vi "PicoScope2000aExampleStreaming.vi"() -> ()   [LabVIEW 2016]
uses:
  Program Files/Pico Technology/SDK/lib/ps2000a.dll
  <vilib>/Waveform/DWDTOps.llb/DWDT Analog to Digital.vi
panel:
  out "Channel A":waveform(dbl)(graph)={"t0"=timestamp(0 s since 1904-01-01), "dt"=1.0000000130088963e-06, "Y"=array[49152 elements]}
  in  "Port 0 Settings":cluster{"Enabled":bool, "Logic Level":i16}={"Enabled"=FALSE, "Logic Level"=9830} {"Logic Level" items=["1.5V TTL"=9830, "2.5V CMOS"=16383]}
  out "Port 0":digitalwaveform(graph)={"t0"=timestamp(0 s since 1904-01-01), "dt"=1.0000000130088963e-06, "Y"={"transitions"=[], "data"=[]}}
  out "Sample Interval (sec)":dbl=1.0000000130088963e-06 format="%#.5p"
  out "Total Samples":u32=3096576 format="%#.6p"
  out "Triggered":bool
  out "TriggeredAt (Total samples)":u32 format="%#.6p"
  out "TriggeredAt (In Buffer)":u32 format="%#.6p"
  in  "Channel A Settings":T1={"Enabled"=TRUE, "Coupling"=1, "Range"=7, "Analogue Offset"=0.0} {"Range" items=["20 mV"=1, "50 mV"=2, "100 mV"=3, "200 mV"=4, "500 mV"=5, "1 V"=6, "2 V"=7, "5 V"=8, "10 V"=9, "20 V"=10]; "Coupling" items=["AC", "DC"]}
  in  "Trigger Settings":T2={"Trigger Enabled"=FALSE, "Trigger Source"=enum."Channel A", "Trigger Threshold (Volts)"=0.0, "Trigger Direction"=2, "Trigger Delay (samples)"=0, "Auto Trigger Time (ms)"=1000} {"Trigger Direction" items=["Rising"=2, "Falling"=3]}
  in  "Acquisition Settings":T3={"Auto Stop"=FALSE, "Desired Sample Interval"=1, "Pre-trigger Samples"=50000, "Post-trigger Samples"=50000, "Down-Sample Ratio"=1, "Down-Sample Mode"=0, "Overview Buffer Size"=1000000, "Time Units"=3} {"Time Units" items=["Nanoseconds (ns)"=2, "Microseconds (us)"=3, "Milliseconds (ms)"=4, "Seconds (s)"=5]; "Overview Buffer Size" format="%.0p"; "Down-Sample Mode" items=["None"=0, "Aggregate"=1, "Average"=2, "Decimate"=4, "Distribution"=8]; "Post-trigger Samples" format="%.0p"; "Pre-trigger Samples" format="%.0p"}
  in  "Apply Settings":bool
  in  "stop":bool
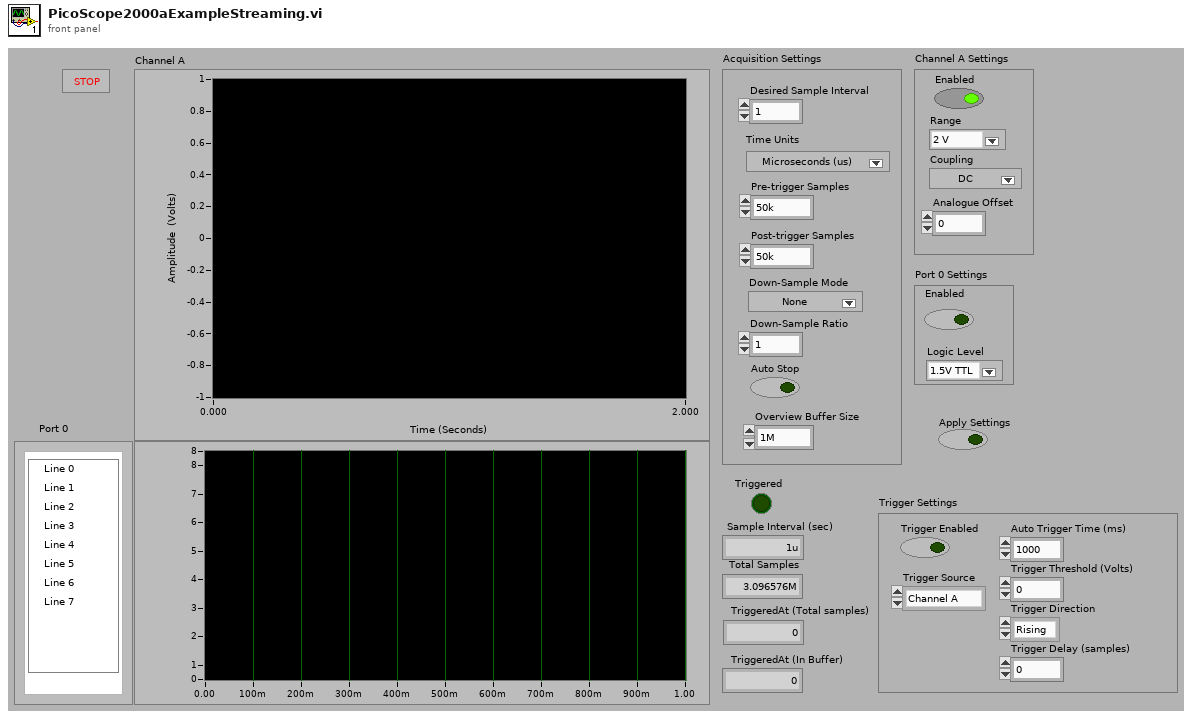
[diagram p1: front panel]
types:
  T1 = cluster{"Enabled":bool, "Coupling":i16, "Range":u16, "Analogue Offset":sgl}
  T2 = cluster{"Trigger Enabled":bool, "Trigger Source":enum16{"Channel A", "Channel B", "Channel C", "Channel D", "Ext."}, "Trigger Threshold (Volts)":dbl, "Trigger Direction":u16, "Trigger Delay (samples)":u32, "Auto Trigger Time (ms)":i16}
  T3 = cluster{"Auto Stop":bool, "Desired Sample Interval":u32, "Pre-trigger Samples":u32, "Post-trigger Samples":u32, "Down-Sample Ratio":u32, "Down-Sample Mode":u32, "Overview Buffer Size":i32, "Time Units":u32}
  T4 = cluster{"Driver Version":string, "USB Version":string, "Hardware":string, "Variant":string, "Batch and Serial":string, "Cal Date":string, "Kernel Version":string, "Digital HW Version":string, "Analogue HW Version":string, "Firmware 1":string, "Firmware 2":string, "MSO":bool, "Number of Channels":i16}
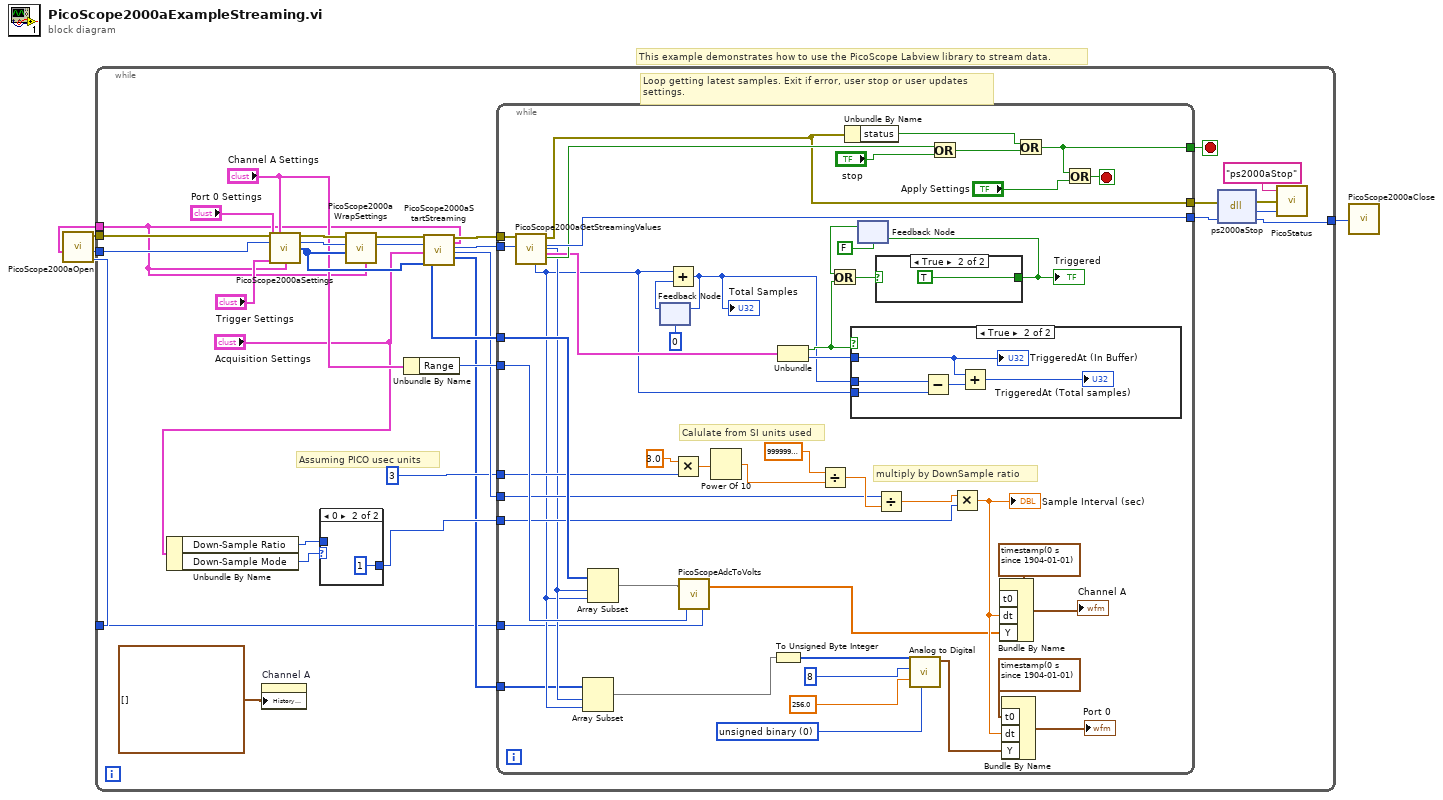
[diagram p0: block diagram]
diagram:
  # "This example demonstrates how to use the PicoScope Labview library to stream data."
  n1 = call "PicoScope2000aOpen.vi"() -> ("Max Adc value"=w4:i16, "handle"=w3:i16, "error out"=w2:errorcluster, "Device Info"=w1:T4)  [unwired: 4 in]
  n2 = while {
    tunnel: [w13] -> w5
    tunnel: w4 -> [w10]
    tunnel: w3 -> [w9]
    tunnel: w2 -> [w8]
    tunnel: w1 -> [w7]
    stop <- w25 stop-if-true
    # "Loop getting latest samples. Exit if error, user stop or user updates \nsettings."
    # "Assuming PICO usec units"
    n3 = Unbundle By Name("Acquisition Settings") -> ("Down-Sample Ratio"=w21:u32, "Down-Sample Mode"=w22:u32)
    n4 = property on="Channel A" class="WFChart (strict)"("History Data"=waveform(dbl)[] []) -> ()  [unwired: 2 in, 2 out]
    n5 = call "PicoScope2000aSettings.vi"("error in"=w8, "Channel A Settings"="Channel A Settings", "handle in"=w9, "Trigger Settings"="Trigger Settings", "Port 0 Settings"="Port 0 Settings", "Device Info"=w7) -> ("error out"=w33:errorcluster, "handle out"=w32:i16, "Enabled Array"=w29:i16[])  [unwired: 7 in]
    n6 = case shown="0" w22 {
      tunnel: [w37 u32 1 ("Down-Sample Ratio")] -> w20
      tunnel: w21 -> [w37 _]
      frame Default {
      }
      frame 0 {
      }
    }
    n7 = call "PicoScope2000aWrapSettings.vi"("Device Info"=w7, "Enabled array"=w29, "Handle In"=w32, "error in (no error)"=w33) -> ("Handle Out"=w30:i16, "error out"=w31:errorcluster)  [unwired: 6 in]
    n8 = Unbundle By Name("Channel A Settings") -> ("Range"=w28:u16)
    n9 = call "PicoScope2000aStartStreaming.vi"("error in"=w31, "handle in"=w30, "Acquisition Settings"="Acquisition Settings", "Enabled Array"=w29, "Device Info"=w7) -> ("Channel A"=w36:i16[], "error out"=w34:errorcluster, "handle out"=w35:i16, "Sample Interval"=w24:u32, "Port 0"=w18:i16[])  [unwired: 10 out]
    n10 = while {
      tunnel: [w82] -> w11
      tunnel: [w85] -> w25
      tunnel: w36 -> [w83]
      tunnel: w35 -> [w81]
      tunnel: w34 -> [w80]
      tunnel: w28 -> [w76]
      tunnel: w24 -> [w59]
      tunnel: u32 3 ("y") -> [w58]
      tunnel: w20 -> [w57]
      tunnel: w18 -> [w46]
      tunnel: [w43] -> w12
      tunnel: w10 -> [w41]
      stop <- w84 stop-if-true
      w54 = u16 0 items=["unsigned binary", "offset binary", "2's complement"] ("data format (offset binary)")
      # "Calulate from SI units used"
      # "multiply by DownSample ratio"
      n11 = call "PicoScope2000aGetStreamingValues.vi"("handle in"=w81, "error in"=w80) -> ("Start Index"=w49:u32, "Trigger"=w74:cluster{bool, "triggeredAt":u32}, "handle out"=w82:i16, "error out"=w43:errorcluster, "Number of Samples"=w48:i32, "Auto Stopped"=w79:bool)  [unwired: 4 in]
      n12 = Array Subset(array=w46, index=w49, length=w48) -> (w47:i16[])
      n13 = Array Subset(array=w83, index=w49, length=w48) -> (w44:i16[])
      n14 = feedback #1(u32 0) -> (w66:u32)
      n15 = Add(x=w48, y=w66) -> (x+y=w67:u32)
      "Total Samples" <- w67
      n16 = feedback-in #1(w67) -> ()
      n17 = Multiply(x=3.0, y=w58) -> (x*y=w61:dbl)
      n18 = call "PicoScopeAdcToVolts.vi"("Max_adc"=w41, "Range Index"=w76, "Data"=w44) -> ("Data"=w40:dbl[])
      n19 = Power Of 10(x=w61) -> (10^x=w62:dbl)
      n20 = To Unsigned Byte Integer(number=w47) -> (unsigned 8bit integer=w50:u8[])
      n21 = Unbundle(w74) -> (w70:bool, "triggeredAt"=w75:u32)
      n22 = Divide(x=sgl 1000000000000000.0 ("y"), y=w62) -> (x/y=w63:dbl)
      n23 = Unbundle By Name(w43) -> ("status"=w87:bool)
      n24 = case shown="True" w70 {
        tunnel: w48 -> [_ w90]
        tunnel: w67 -> [_ w94]
        tunnel: w75 -> [_ w92]
        frame False {
        }
        frame True {
          n25 = Subtract(x=w94, y=w90) -> (x-y=w93:u32)
          n26 = Add(x=w92, y=w93) -> (x+y=→"TriggeredAt (Total samples)":u32)
          "TriggeredAt (In Buffer)" <- w92
        }
      }
      n27 = feedback #2(FALSE) -> (w69:bool)
      n28 = Or(x=w69, y=w70) -> (x .or. y?=w72:bool)
      n29 = case shown="True" w72 {
        selector: w72 -> [w88 _]
        tunnel: [w88 TRUE] -> w71
        frame False {
        }
        frame True {
        }
      }
      "Triggered" <- w71
      n30 = feedback-in #2(w71) -> ()
      n31 = Divide(x=w59, y=w63) -> (x/y=w60:dbl)
      n32 = call-poly <vilib>:"Analog to Digital.vi"("data format (offset binary)"=w54, "full-scale range (pk-pk)"=256.0, "resolution (16 bit)"=8, "analog waveform"=w50) -> ("digital waveform"=w51:digitalwaveform)  [unwired: 4 in, 3 out]
      n33 = Or(x=w79, y="stop") -> (x .or. y?=w77:bool)
      n34 = Multiply(x=w60, y=w57) -> (x*y=w45:dbl)
      "Sample Interval (sec)" <- w45
      n35 = Bundle By Name("t0"=timestamp(0 s since 1904-01-01), "dt"=w45, "Y"=w40) -> (→"Channel A":waveform(dbl))  [unwired: 1 in]
      n36 = Bundle By Name("t0"=timestamp(0 s since 1904-01-01), "dt"=w45, "Y"=w51) -> (→"Port 0":digitalwaveform)  [unwired: 1 in]
      n37 = Or(x=w87, y=w77) -> (x .or. y?=w85:bool)
      n38 = Or(x=w85, y="Apply Settings") -> (x .or. y?=w84:bool)
    }
    n39 = dll-call lib="/////Program Files/Pico Technology/SDK/lib/PS2000a.dll" fn="ps2000aStop"(error in=w12, "handle"=w11) -> (error out=w16:errorcluster, "PICO_STATUS"=w15:u32, "handle"=w13:i16)  [unwired: 2 in, 1 out]
    n40 = call "PicoStatus.vi"("PICO STATUS"=w15, "error in"=w16, "source"="ps2000aStop") -> ()  [unwired: 1 out]
  }
  n41 = call "PicoScope2000aClose.vi"("handle"=w5) -> ()
